vi "Bordeaux to Botpose Convert Coordinates.vi"(11 "Pos In":cluster{"x":dbl, "y":dbl}) -> (3 "Pos Out":cluster{dbl, dbl})   [LabVIEW 2025]
panel:
  out "new x":dbl
  out "new y":dbl
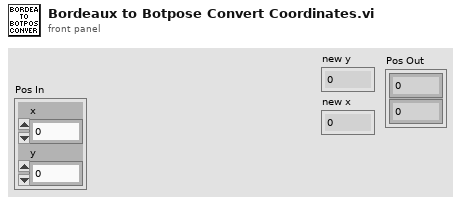
[diagram p1: front panel]
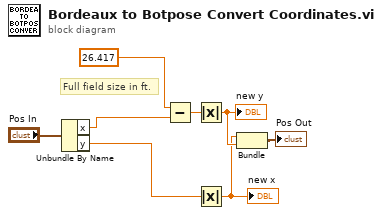
[diagram p0: block diagram]
diagram:
  # "Full field size in ft."
  n1 = Unbundle By Name("Pos In") -> ("x"=w6:dbl, "y"=w4:dbl)
  n2 = Subtract(x=26.417, y=w6) -> (x-y=w7:dbl)
  n3 = Absolute Value(x=w7) -> (abs(x)=w2:dbl)
  "new y" <- w2
  n4 = Absolute Value(x=w4) -> (abs(x)=w1:dbl)
  "new x" <- w1
  n5 = Bundle(w1, w2) -> (→"Pos Out":cluster{dbl, dbl})  [unwired: 1 in]
